vi "Query.vi"(8 "error in":errorcluster, 10 "Query":string, 11 "DB-Engine in":refnum<class "DB-Interface.lvclass">) -> (0 "error out":errorcluster, 1 "Meta Data":variant, 2 "Return Data":string[][](array[string]), 3 "DB-Engine out":refnum<class "DB-Interface.lvclass">, 4 "Field Names":string[](array[string]))   [LabVIEW 2014, in "hse-db.lvlib" / "DB-Interface.lvclass"]
uses:
  DB-Interface.lvclass
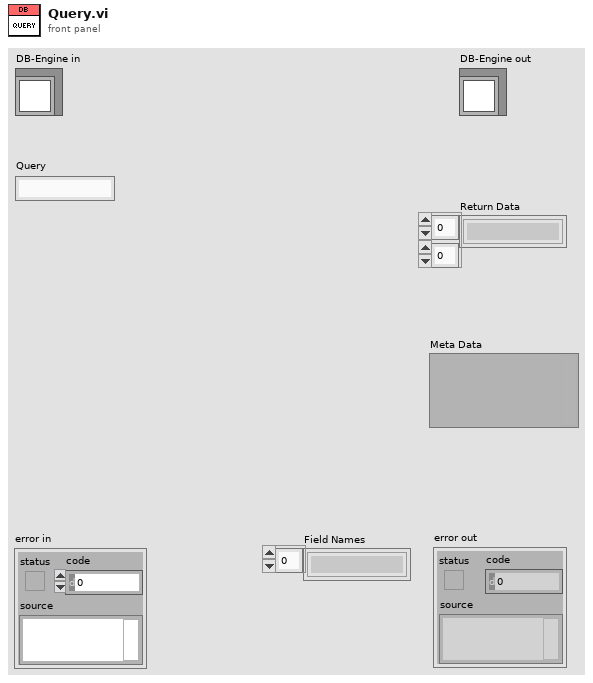
[diagram p1: front panel]
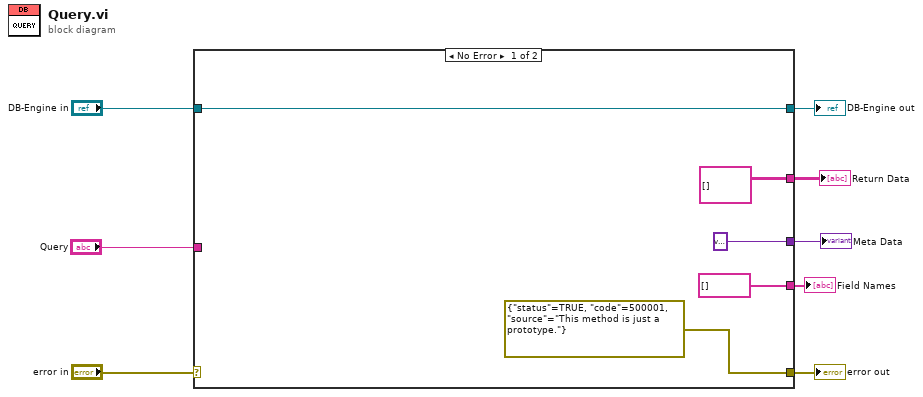
[diagram p0: block diagram]
diagram:
  n1 = case shown="No Error" "error in" {
    selector: "error in" -> [_ w15]
    tunnel: [errorcluster {"status"=TRUE, "code"=500001, "source"="This method is just a prototype."} ("error IO") w15] -> w7
    tunnel: [w13 w14] -> w5
    tunnel: "DB-Engine in" -> [w13 w14]
    tunnel: "Query" -> [_ _]
    tunnel: [string[][] [] _] -> w2
    tunnel: [variant _] -> w3
    tunnel: [string[] [] _] -> w1
    frame No Error {
    }
    frame Error {
    }
  }
  "error out" <- w7
  "DB-Engine out" <- w5
  "Meta Data" <- w3
  "Return Data" <- w2
  "Field Names" <- w1
